vi "TcpWriteRead.vi"(8 "error in":errorcluster, 9 "port":u16=9999, 10 "address":string, 11 "data in":string="SAY_HELLO_WOLRD") -> (0 "error out":errorcluster, 3 "data out":string)   [LabVIEW 2018]
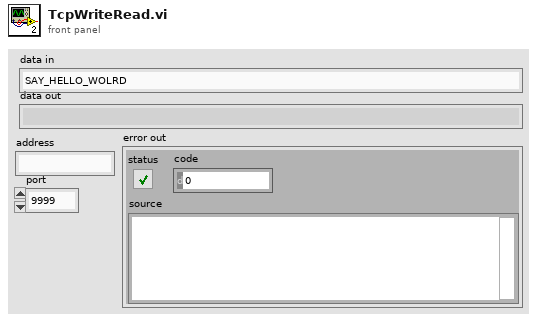
[diagram p1: front panel]
types:
  T1 = enum16{"Standard", "Buffered", "CRLF", "Immediate"}
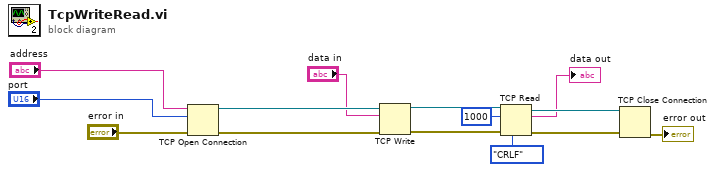
[diagram p0: block diagram]
diagram:
  n1 = TCP Open Connection(address="address", remote port or service name="port", error in (no error)="error in") -> (connection ID=w14:refnum<k5>, error out=w3:errorcluster)  [unwired: 2 in]
  n2 = TCP Write(connection ID=w14, data in="data in", error in (no error)=w3) -> (connection ID out=w13:refnum<k5>, error out=w6:errorcluster)  [unwired: 1 in, 1 out]
  n3 = TCP Read(connection ID=w13, bytes to read=1000, error in (no error)=w6, 7:T1."CRLF" ("mode (standard)")) -> (connection ID out=w12:refnum<k5>, data out=→"data out":string, error out=w2:errorcluster)  [unwired: 1 in]
  n4 = TCP Close Connection(connection ID=w12, error in (no error)=w2) -> (error out=→"error out":errorcluster)  [unwired: 1 in, 1 out]
